vi "FPGA DMA Top.vi"() -> ()   [LabVIEW 2017]
uses:
  <vilib>/Platform/TimedLoop/XDataNode/timing_clust.ctl
  <vilib>/Platform/TimedLoop/XDataNode/nitl_modes.ctl
  <vilib>/Platform/TimedLoop/XDataNode/wakeup.ctl
  <vilib>/rvi/Emulation/niFpgaGetClockAttributes.vi
  <vilib>/rvi/Emulation/niFpgaSctlEmulationGetInTimedLoop.vi
  <vilib>/rvi/Emulation/niFpgaEmulationReportErrorSimple.vi
  <vilib>/rvi/Emulation/niFpgaEmulationIsFPGAContextNoSignature.vi
  <vilib>/rvi/errors/niFpgaSetErrorForExecOnDevCompSimple.vi
  <vilib>/rvi/eio/common/nirviEmuReportErrorAndStop.vi
  <vilib>/rvi/DataTransferAndStorage/Container/Common/niFpgaContainerGetUniqueNameForEmu.vi
  <vilib>/rvi/FIFO/Fifo_Resource/nirvififoEmulationSetSize.vi
  <vilib>/rvi/FIFO/Fifo_Resource/nirviFifoEmulationQueueMgr.vi
  <instcachedir>/0/nirviFifoEmulationQueueMgr_E5CAEC123FF24DC58D834DCA3CDAA9B5.lvgen/nirviFifoEmulationQueueMgr_E5CAEC123FF24DC58D834DCA3CDAA9B5_000.vi
  <vilib>/rvi/FIFO/Fifo_Resource/nirvififoEmulationDetermineInputValidOut.vi
  <vilib>/rvi/FIFO/Fifo_Resource/nirvififoEmulationCreateLock.vi
  <vilib>/rvi/Emulation/niFpgaProcessEmulError.vi
  <vilib>/rvi/FIFO/Fifo_Resource/nirvififoEmulationObtainLock.vi
  <vilib>/rvi/FIFO/Fifo_Resource/nirvififoEmulationReleaseLock.vi
  <vilib>/rvi/occurrence/nirviWaitOnOccurrenceBase.vi
  <vilib>/rvi/errors/nirviReportUnexpectedCaseInternalError.vi
  <vilib>/rvi/errors/nirviReportUnexpectedCaseInternalError (U32).vi
  <vilib>/rvi/Emulation/niFpgaCriticalErrorInLSC.vi
  <vilib>/Utility/error.llb/Clear Errors.vi
  <vilib>/rvi/interface/RandomDataEmulation/niFpgaRandomDataHandleErrors.vi
  <vilib>/rvi/DataTransferAndStorage/Container/XNode/niFpgaContainer.xnode
  <vilib>/rvi/FIFO/Fifo_Resource/nirvififoEmulationWrite.vi
  <vilib>/Platform/TimedLoop/XDataNode/XDataNode.xnode
  <vilib>/rvi/FIFO/Fifo_Resource/nirvififoEmulationRead.vi
  <vilib>/rvi/interface/RandomDataEmulation/nirviRandomDataFpgaReadWriteTemplate.vi
  <vilib>/Platform/TimedLoop/XDataNode/XDNodeRunTimeDep.lvlib
panel:
  out "sgl_out":sgl
  in  "sgl_in":sgl
  out "int_out":u32
  in  "int_in":u32
  out "bool_out":bool
  in  "bool_in":bool
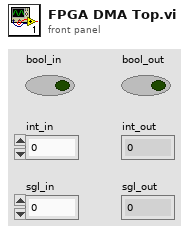
[diagram p1: front panel]
types:
  T1 = typedef "XDNodeRunTimeDep.lvlib/timing_clust.ctl" = cluster{"Expected End [f-1]":u64, "Actual End [f-1]":u64, "Finished Late? [f-1]":bool, "Expected End [i-1]":u64, "Actual End [i-1]":u64, "Finished Late? [i-1]":bool, "Expected Start [i]":u64, "Actual Start [i]":u64, "Expected Start [f]":u64, "Actual Start [f]":u64, "Source Name":string, "Structure Name":string, "Period":i64, "Deadline":i64, "Offset":i64, "Start":i64, "Priority":i32, "Timeout":i32, "Mode":T2, "Wakeup Reason":T3, "Error":errorcluster, "Source Type":string, "Secondary Source Type":string, "Global End Time":u64, "Global Start Time":u64, "Frame Duration":u64, "Iteration Duration":u64, "Assigned CPU":i32, "I/O Scan Engine Mode":u32}
  T2 = typedef "XDNodeRunTimeDep.lvlib/nitl_modes.ctl" = enum32{"No Change", "Process missed periods, maintain original phase", "Discard missed periods, maintain original phase", "Process missed periods, ignore original phase", "Discard missed periods, ignore original phase"}
  T3 = typedef "XDNodeRunTimeDep.lvlib/wakeup.ctl" = enum32{"Normal", "Aborted", "Asynchronous wakeup", "Timing source error", "Timed loop error", "Timeout"}
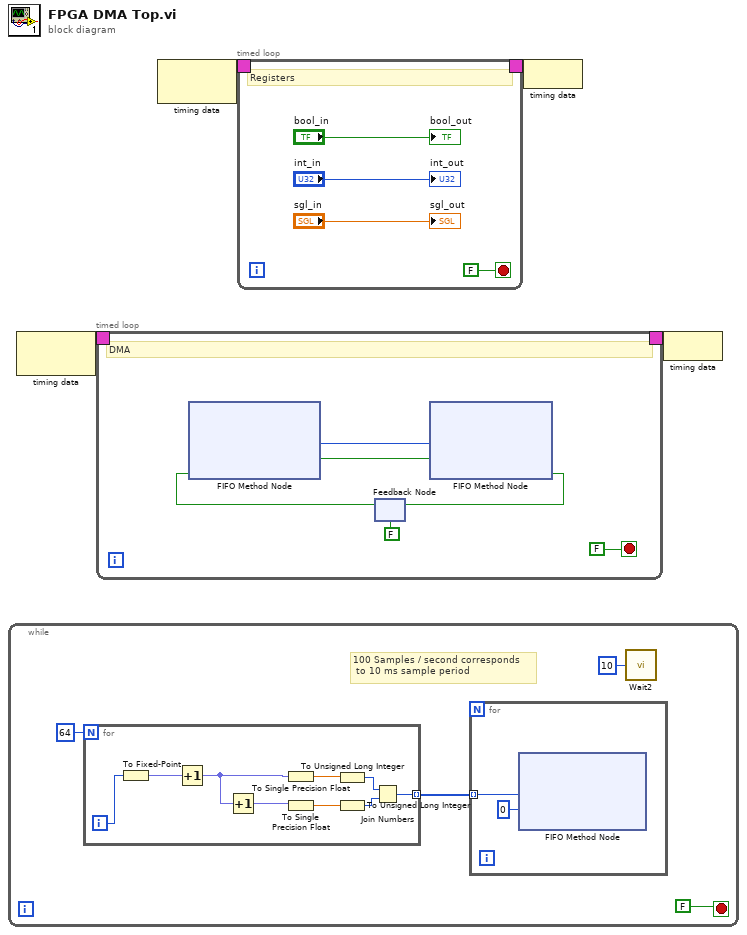
[diagram p0: block diagram]
diagram:
  n1 = while {
    stop <- FALSE stop-if-true
    # "100 Samples / second corresponds\n to 10 ms sample period"
    n2 = for {
      N: 64 -> [_]
      tunnel: [w9] -> w7 mode=indexing
      i -> [w12]
      n3 = To Fixed-Point(number=w12) -> (fixed-point=w13:fxp<+/-,32,32>)  [unwired: 1 in]
      n4 = Increment(x=w13) -> (x+1=w11:fxp<+/-,33,33>)
      n5 = Increment(x=w11) -> (x+1=w10:fxp<+/-,33,33>)
      n6 = To Single Precision Float(number=w11) -> (single precision float=w17:sgl)
      n7 = To Single Precision Float(number=w10) -> (single precision float=w16:sgl)
      n8 = To Unsigned Long Integer(number=w17) -> (unsigned 32bit integer=w14:u32)
      n9 = To Unsigned Long Integer(number=w16) -> (unsigned 32bit integer=w15:u32)
      n10 = Join Numbers(hi=w14, lo=w15) -> ((hi.lo)=w9:u64)
    }
    n11 = for {
      tunnel: w7 -> [w19] mode=indexing
      n12 = xnode ("FIFO Method Node")("Element"=w19, "Timeout"=0) -> ()  [unwired: 1 in, 2 out]
    }
    n13 = call "Wait2"("Count(mSec)"=u32 10) -> ()  [unwired: 1 out]
  }
  n14 = node-c288() -> (w2:T1)  [unwired: 1 in]
  n15 = timed-loop {
    timing: w2 -> [_]
    timing-out: [_] -> w1
    stop <- FALSE stop-if-true
    # "DMA"
    n16 = feedback #1(FALSE ("Ready for Input")) -> (w22:bool)
    n17 = xnode ("FIFO Method Node")("Ready for Output"=w22) -> ("Element"=w24:u64, "Output Valid"=w20:bool)  [unwired: 1 in, 1 out]
    n18 = xnode ("FIFO Method Node")("Element"=w24, "Input Valid"=w20) -> ("Ready for Input"=w23:bool)  [unwired: 1 in, 1 out]
    n19 = feedback-in #1(w23) -> ()
  }
  n20 = node-c288() -> (w4:T1)  [unwired: 1 in]
  n21 = timed-loop {
    timing: w4 -> [_]
    timing-out: [_] -> w3
    stop <- FALSE stop-if-true
    # "Registers"
    "bool_out" <- "bool_in"
    "int_out" <- "int_in"
    "sgl_out" <- "sgl_in"
  }
  n22 = node-c288(w3) -> ()
  n23 = node-c288(w1) -> ()
